vi "AddProject.vi"(8 "error in (no error)":errorcluster, 9 "NewProjectName":string, 11 "Project.lvclass In":refnum<class "Project.lvclass">) -> (0 "error out":errorcluster, 2 "ProjectSelectIdx":i32, 3 "Project.lvclass Out":refnum<class "Project.lvclass">)   [LabVIEW 2014, in "Project.lvclass"]
uses:
  Project.lvclass
  StepSetupDataTypeDefine.ctl
  StepData/Control/AllStepTypeData.ctl
  StepData/Control/StepTypeEnum.ctl
  StepData/Control/MoveData.ctl
  StepData/Control/MeasureData.ctl
  Project.lvclass/Project.ctl
  StepData/StepData.lvclass
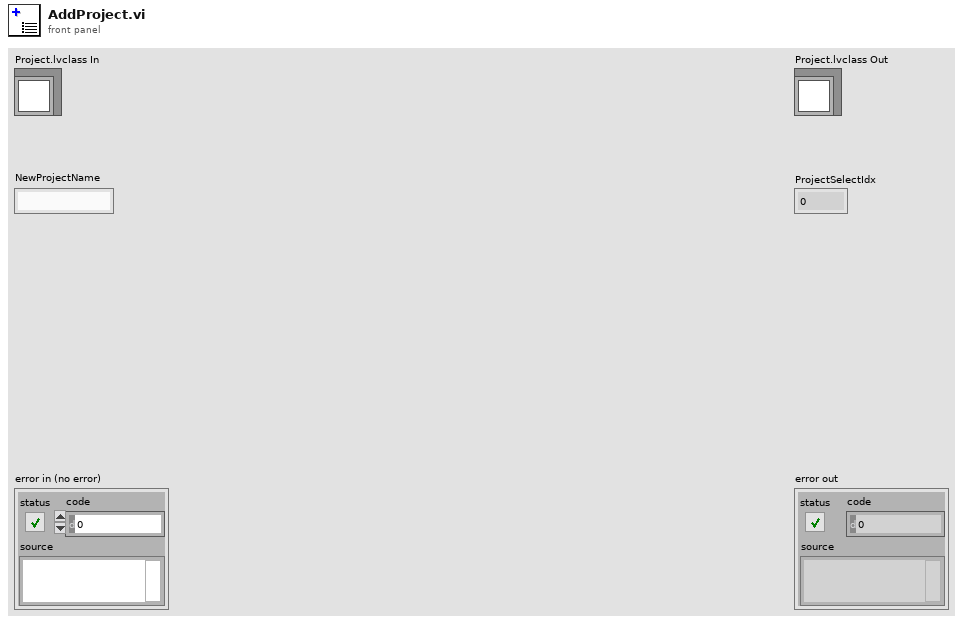
[diagram p1: front panel]
types:
  T1 = typedef "Project.lvclass/StepSetupDataTypeDefine.ctl" = cluster{"AllStepTypeData":T2}[]
  T2 = typedef "StepData.lvclass/AllStepTypeData.ctl" = cluster{"StepName":string, "StepTypeEnum":T3, "MoveData":T4, "MeasureData":T5}
  T3 = typedef "StepData.lvclass/StepTypeEnum.ctl" = enum16{"Move", "Measure"}
  T4 = typedef "StepData.lvclass/MoveData.ctl" = cluster{"Axis":u16, "Position":dbl, "Speed":dbl, "Acc/Dec":dbl, "Mode":u16}
  T5 = typedef "StepData.lvclass/MeasureData.ctl" = cluster{"Sensor No.":i32, "Log?":bool}
  T6 = typedef "Project.lvclass/ProjectDataTableTypeDefine.ctl" = string[][]
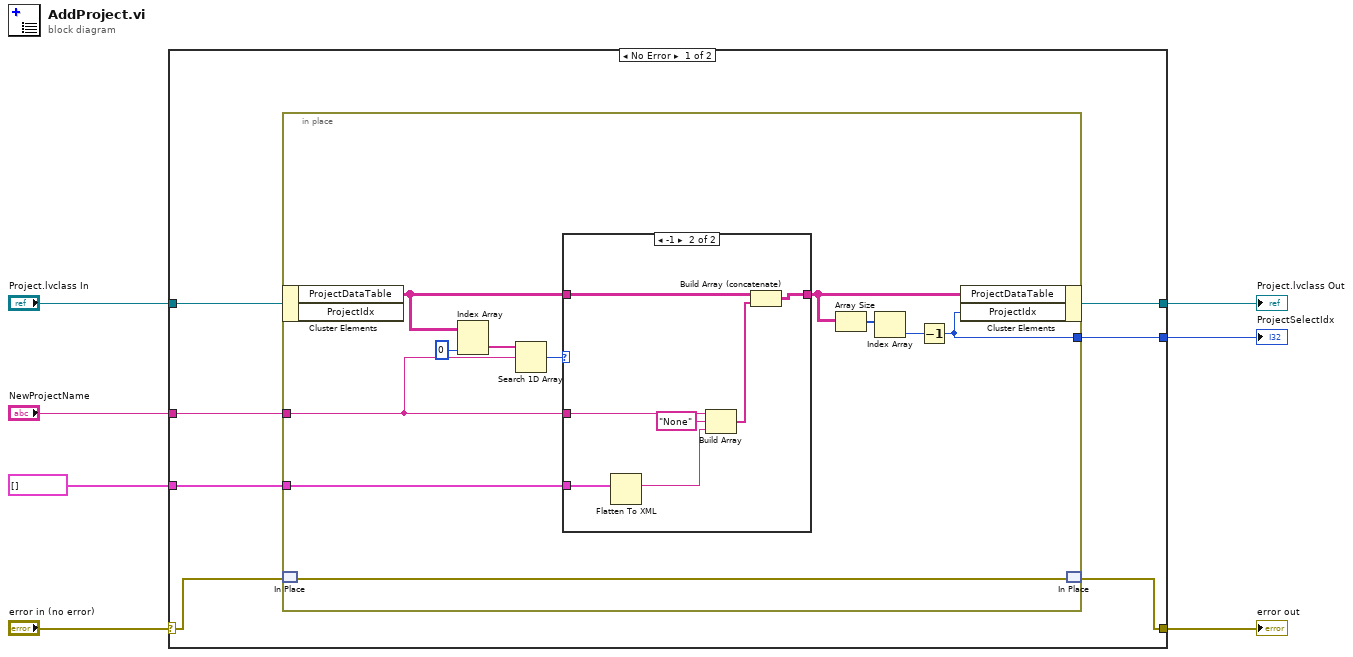
[diagram p0: block diagram]
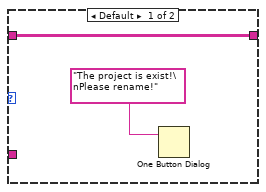
[diagram p2: hidden frame]
diagram:
  n1 = case shown="No Error" "error in (no error)" {
    selector: "error in (no error)" -> [w13 w36]
    tunnel: [w11 w36] -> w6
    tunnel: "Project.lvclass In" -> [w14 w35]
    tunnel: "NewProjectName" -> [w12 _]
    tunnel: [w10 w35] -> w3
    tunnel: [w9 _] -> w2
    tunnel: T1 [] ("StepSetupClusterArray") -> [w8 _]
    frame No Error {
      n2 = in-place {
        in-place-border: w12 -> [w21]
        in-place-border: [w16] -> w9
        in-place-border: w8 -> [w15]
        n3 = in-place-cluster #1(w14) -> ("ProjectDataTable"=w22:T6)  [unwired: 1 out]
        n4 = in-place-match #2(w13) -> (w17:errorcluster)
        n5 = Index Array(array=w22, index (col)=0 ("disabled index (col)")) -> (element=w24:string[])  [unwired: 1 in]
        n6 = Search 1D Array(1D array=w24, element=w21) -> (index of element=w23:i32)  [unwired: 1 in]
        n7 = case shown="-1" w23 {
          tunnel: w22 -> [w27 w34]
          tunnel: w21 -> [_ w33]
          tunnel: [w27 w31] -> w18
          tunnel: w15 -> [_ w29]
          frame Default {
            n8 = One Button Dialog(message="The project is exist!\nPlease rename!") -> ()  [unwired: 1 in, 1 out]
          }
          frame -1 {
            n9 = Flatten To XML(anything=w29) -> (xml string=w28:string)
            n10 = Build Array(w33, "None" ("element"), w28) -> (w32:string[])
            n11 = Build Array (concatenate)(w34, w32) -> (w31:T6)
          }
        }
        n12 = Array Size(array=w18) -> (size(s)=w20:i32[])
        n13 = Index Array(array=w20) -> (element=w19:i32)  [unwired: 1 in]
        n14 = Decrement(x=w19) -> (x-1=w16:i32)
        n15 = in-place-cluster #1("ProjectDataTable"=w18, "ProjectIdx"=w16) -> (w10:refnum<class "Project.lvclass">)
        n16 = in-place-match #2(w17) -> (w11:errorcluster)
      }
    }
    frame Error {
    }
  }
  "error out" <- w6
  "Project.lvclass Out" <- w3
  "ProjectSelectIdx" <- w2
